vi "Measurement UI.vi"() -> ()   [LabVIEW 2021, in "Single Point_Channel Ganging_UI.lvlib"]
uses:
  Single Point_Channel Ganging_UI.lvlib
  shared/UI/controls/view.ctl
panel:
  in  "MeasGraphs":enum32{"Results", "Hidden Controls"}(tab)
  in  "Current v/s Time":string="CURRENT v/s TIME"
  in  "Voltage v/s Time":string="VOLTAGE v/s TIME"
  in  "view current legend":T1
  in  "view voltage legend":T1
  out "CurrentGraph":waveform(dbl)[](graph) caption="AC"
  out "VoltageGraph":waveform(dbl)[](graph) caption="AC"
  in  "Mode of operation":T2(ring)
  out "Maximum values":dbl[](array[numeric])
  out "Minimum values":dbl[](array[numeric])
  out "Mean values":dbl[](array[numeric])
  in  "Load resource names":string[](array[string])
  in  "Power ON/Source resource names":string[](array[string])
  out "Ganged load currents":dbl[](array[numeric])
  out "Ganged load voltages":dbl[](array[numeric])
  out "Ganged source currents":dbl[](array[numeric])
  out "Ganged source voltages":dbl[](array[numeric])
  out "Load currents":dbl[](array[numeric])
  out "Load voltages":dbl[](array[numeric])
  out "Source currents":dbl[](array[numeric])
  out "Source voltages":dbl[](array[numeric])
  out "dt":dbl[](array[numeric])
  out "Meas Table":string[][](table)=[["Source Voltage (V)"], ["Source Current (A)"], ["Load Voltage (V)"], ["Load Current (A)"]]
  in  "ModeOfConfiguration":T3(tab)
  in  "DEVICE POWER":bool=TRUE
  out "Status":string
  in  "Load config power on":string="Load Config"
  in  "POWERON/OFFLOADResourceNames":refnum<k15>[](array[refnum]) caption="RESOURCE NAMES\n(Single/Master & Slave)"
  in  "Source config power on":string="Source Config"
  in  "POWERON/OFFSOURCEResourceNames":refnum<k15>[](array[refnum]) caption="RESOURCE NAMES\n(Single/Master & Slave)"
  in  "Power on/off source sense":i32(ring)=1009 caption="SENSE" items=["Local"=1008, "Remote"=1009]
  in  "Power on/off Source voltage/current limit range":dbl=20.0 caption="CURRENT LIMIT" format="%#_6pA"
  in  "Power on/off Source voltage/current level":dbl=6.0 caption="VOLTAGE LEVEL" format="%#_6pV"
  in  "Power on/off source system configuration":enum32{"Series", "Parallel"}(ring)=enum."Parallel" caption="SYSTEM CONFIG"
  in  "Power on/off output function":i32(ring)=1006 caption="OUTPUT FUNCTION" items=["DC Voltage"=1006, "DC Current"=1007]
  out "Eload status":string
  in  "MeasConfigurations":T4(tab)=enum."Source Config"
  in  "Measurement timeout":dbl=1.0 caption="MEASUREMENT TIMEOUT" format="%.3ps"
  in  "Aperture time":dbl=0.01666 caption="APERTURE TIME" format="%.3ps"
  in  "Measurement duration":dbl=1.0 caption="MEASUREMENT DURATION" format="%.3ps"
  in  "Source voltage/current compensation frequency":dbl(slide)=3530.0 caption="COMP. FREQUENCY" scale=50.0..1000000.0 scale format="%#_6pHz"
  in  "Source voltage/current pole-zero ratio":dbl(slide)=2.0 caption="POLE-ZERO RATIO" scale=0.0625..16.0
  in  "Source voltage/current gain bandwidth":dbl(slide)=2000.0 caption="GAIN BANDWIDTH" scale=10.0..1000000.0 scale format="%#_6pHz"
  in  "Source enable/disable":bool=TRUE caption="Source Enable/Disable"
  in  "PPSResourceNames":refnum<k15>[](array[refnum]) caption="RESOURCE NAMES\n(Single/Master & Slave)"
  in  "Source transient response":i32(ring)=1038 caption="TRANSIENT RESPONSE" items=["Slow"=1041, "Normal"=1038, "Fast"=1039, "Custom"=1042]
  in  "Power ON/Source sense":i32(ring)=1009 caption="SENSE" items=["Local"=1008, "Remote"=1009]
  in  "Source voltage/current level range":dbl=20.0 caption="VOLTAGE LEVEL RANGE" format="%#_6pV"
  in  "Power ON/Source voltage/current level":dbl=6.0 caption="VOLTAGE LEVEL" format="%#_6pV"
  in  "Source current/voltage limit high":dbl=25.0 caption="CURRENT LIMIT/LIMIT HIGH" format="%#_6pA"
  in  "Power ON/Source current/voltage limit range":dbl=25.0 caption="CURRENT LIMIT RANGE" format="%#_6pA"
  in  "Source limit symmetry":enum32{"Symmetric", "Asymmetric"}(ring)=enum."Asymmetric" caption="LIMIT SYMMETRY"
  in  "Source current/voltage limit low":dbl=-0.6 caption="CURRENT LIMIT LOW" format="%#_6pA"
  in  "Power ON/Source system configuration":enum32{"Series", "Parallel"}(ring)=enum."Parallel" caption="SYSTEM CONFIG"
  in  "Source compliance":string="Compliance"
  in  "Source sourceadapt":string="SourceAdapt"
  in  "Power ON/Source output function":i32(ring)=1006 caption="OUTPUT FUNCTION" items=["DC Voltage"=1006, "DC Current"=1007]
  in  "Load voltage/current compensation frequency":dbl(slide)=3530.0 caption="COMP. FREQUENCY" scale=50.0..1000000.0 scale format="%#_6pHz"
  in  "Load voltage/current pole-zero ratio":dbl(slide)=2.0 caption="POLE-ZERO RATIO" scale=0.0625..16.0
  in  "Load voltage/current gain bandwidth":dbl(slide)=2000.0 caption="GAIN BANDWIDTH" scale=10.0..1000000.0 scale format="%#_6pHz"
  in  "Load device voltage/current rating":dbl=30.0 caption="MAX CURRENT PER LOAD" format="%#_6pA"
  in  "Load sourceadapt":string="SourceAdapt"
  in  "Load compliance":string="Compliance"
  in  "Load system configuration":enum32{"Series", "Parallel"}(ring)=enum."Parallel" caption="SYSTEM CONFIG"
  in  "Load current/voltage limit low":dbl caption="VOLTAGE  LIMIT LOW" format="%#_6pV"
  in  "Load limit symmetry":enum32{"Symmetric", "Asymmetric"}(ring) caption="LIMIT SYMMETRY"
  in  "Load current/voltage limit range":dbl=6.0 caption="VOLTAGE LIMIT RANGE" format="%#_6pV"
  in  "Load current/voltage limit high":dbl=inf caption="VOLTAGE LIMIT/LIMIT HIGH" format="%#_6p"
  in  "Load voltage/current level":dbl=2.0 caption="CURRENT LEVEL" format="%#_6pA"
  in  "Load voltage/current level range":dbl=40.0 caption="CURRENT LEVEL RANGE" format="%#_6pA"
  in  "Load sense":i32(ring)=1009 caption="SENSE" items=["Local"=1008, "Remote"=1009]
  in  "Load transient response":i32(ring)=1038 caption="TRANSIENT RESPONSE" items=["Slow"=1041, "Normal"=1038, "Fast"=1039, "Custom"=1042]
  in  "Load output function":i32(ring)=1007 caption="OUTPUT FUNCTION" items=["DC Voltage"=1006, "DC Current"=1007]
  in  "Load enable/disable":bool=TRUE caption="Load Enable/Disable"
  in  "LoadResourceNames":refnum<k15>[](array[refnum]) caption="RESOURCE NAMES\n(Single/Master & Slave)"
  # "V"
  # "I"
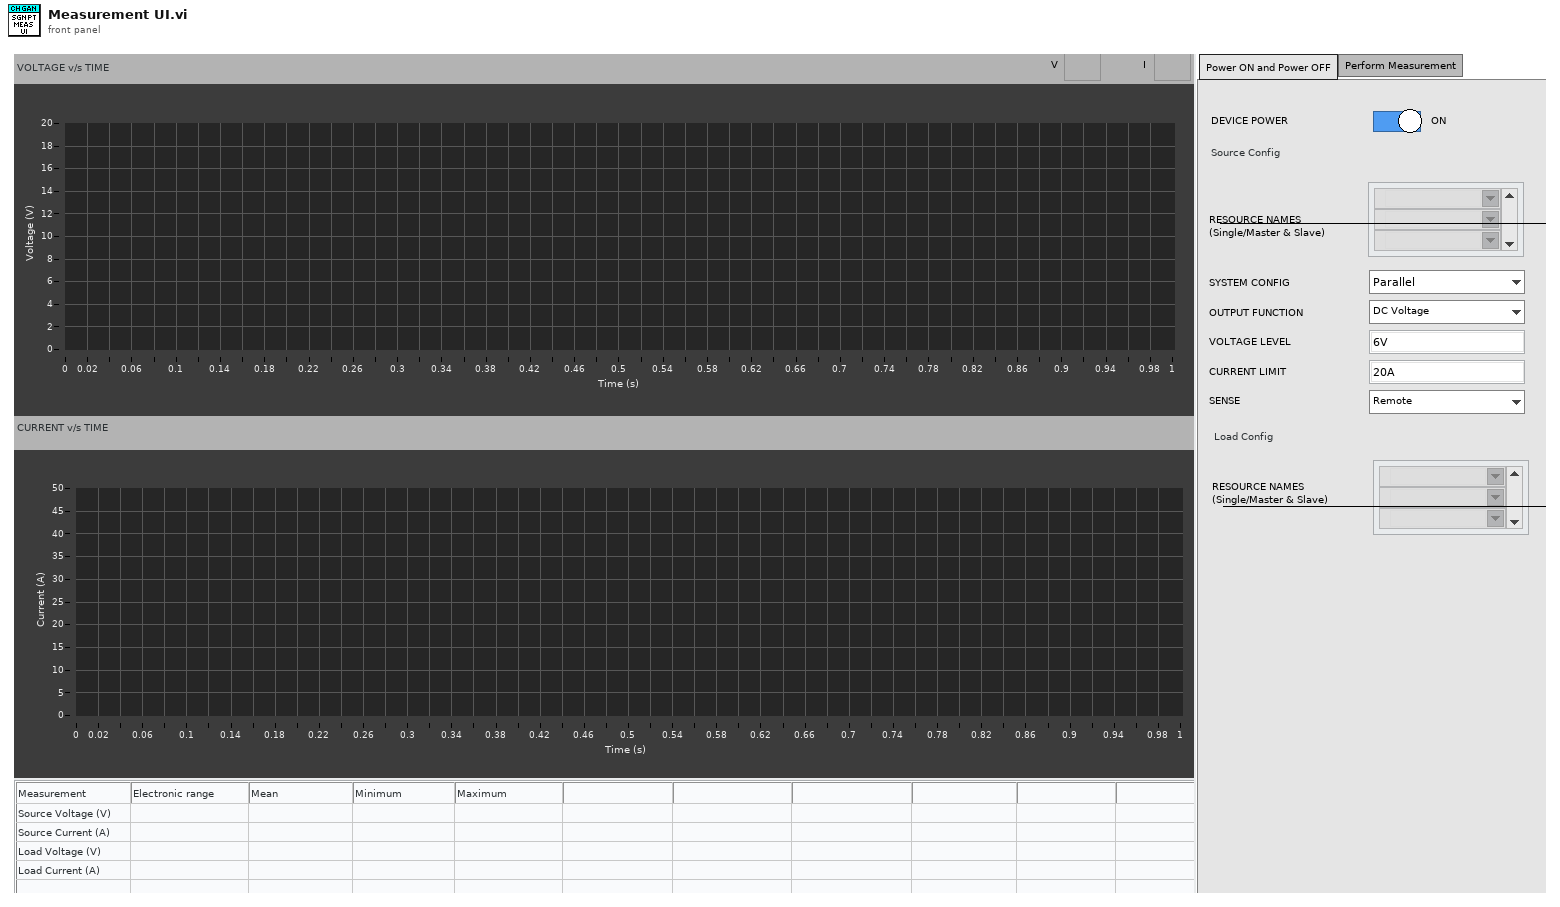
[diagram p1: front panel]
types:
  T1 = typedef "view.ctl" = bool
  T2 = enum32{"Power on the DUT", "Perform measurement", "Power off the DUT"}
  T3 = enum32{"Power ON and Power OFF", "Perform Measurement"}
  T4 = enum32{"Timings", "Source Config", "Load Config"}
  T5 = enum8{"Enabled", "Disabled", "Disabled and Grayed Out"}
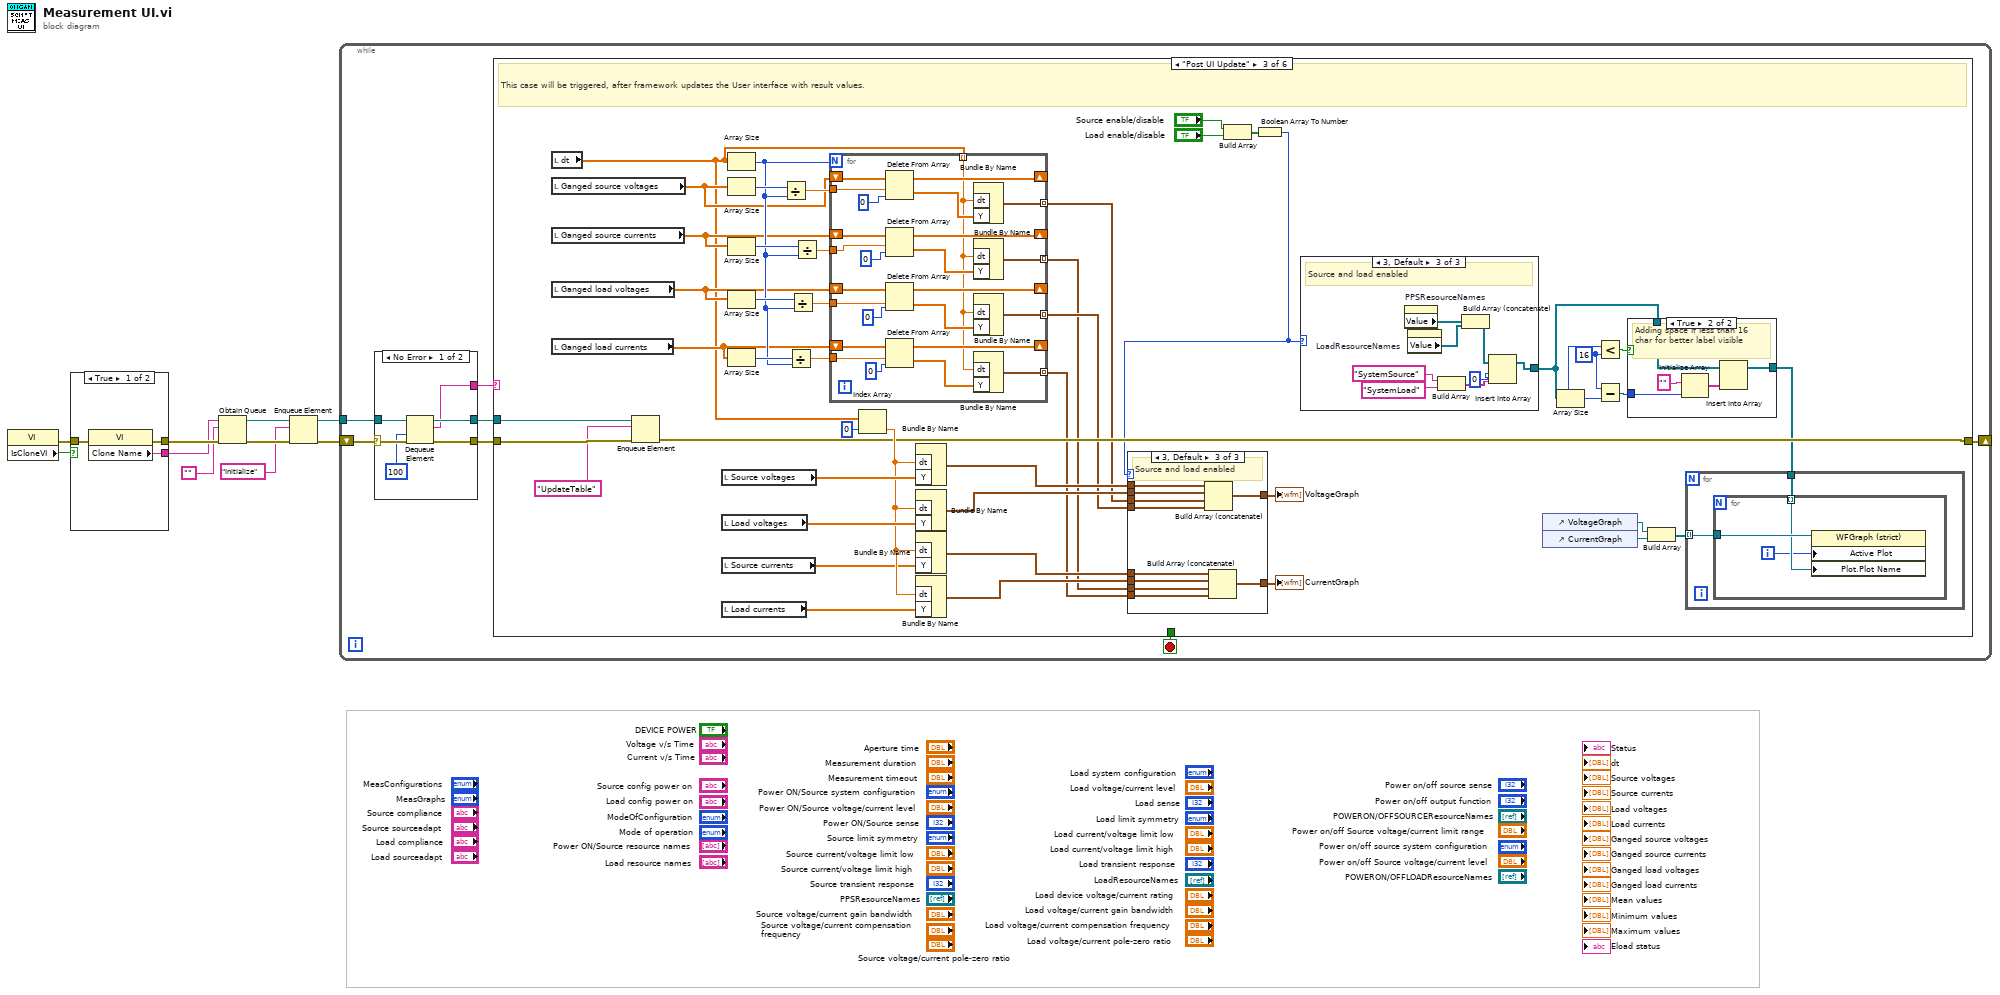
[diagram p0: block diagram]
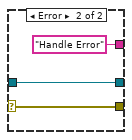
[diagram p2: hidden frame]
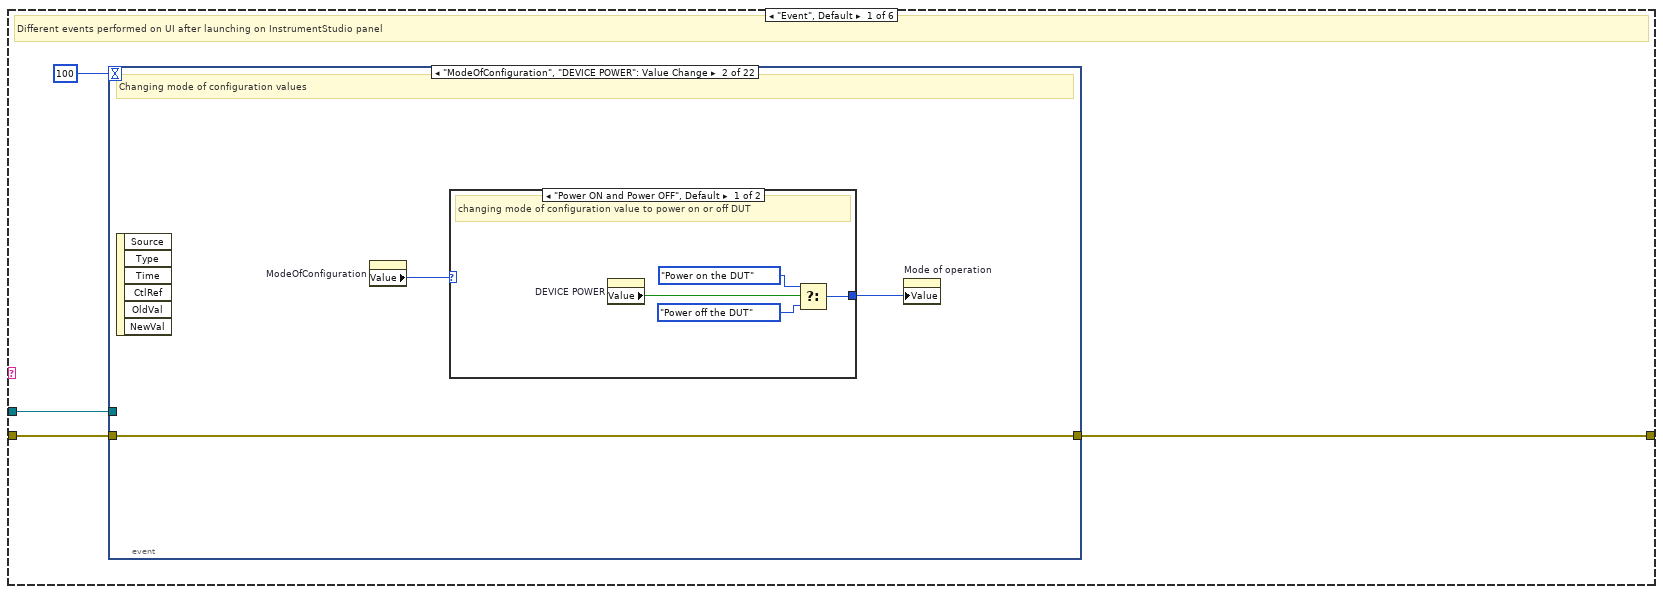
[diagram p3: hidden frame]
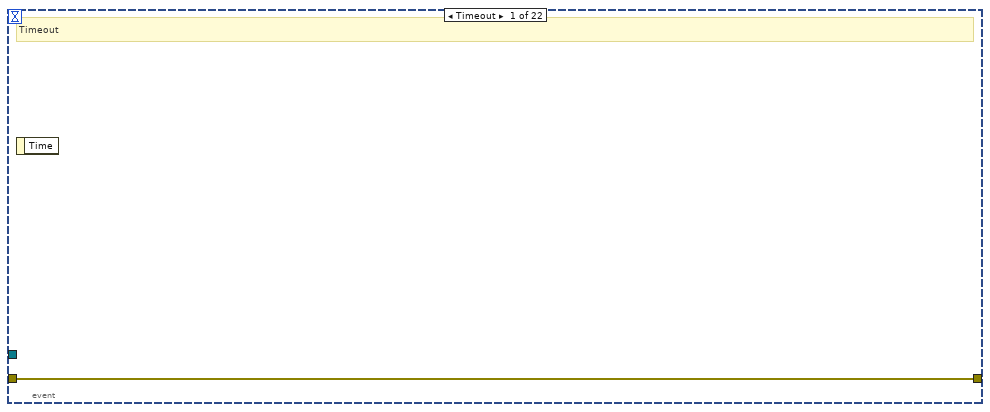
[diagram p4: hidden frame]
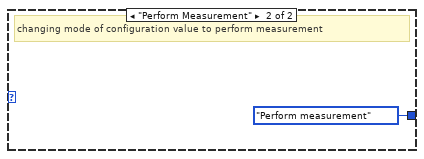
[diagram p5: hidden frame]
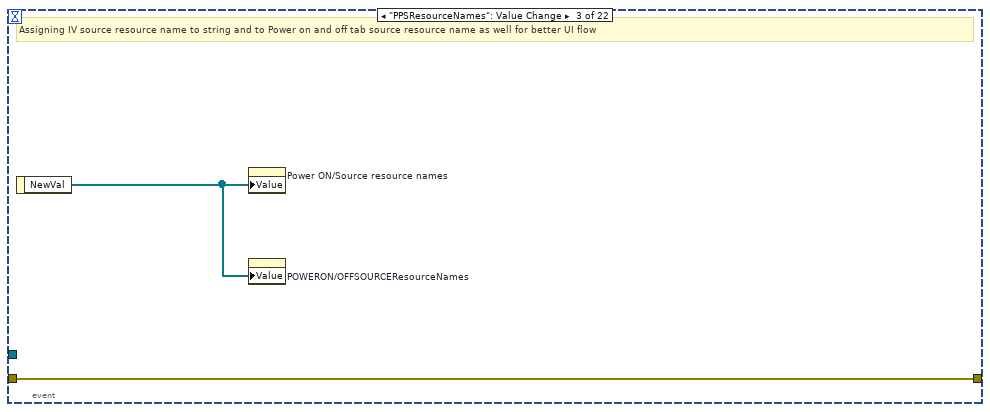
[diagram p6: hidden frame]
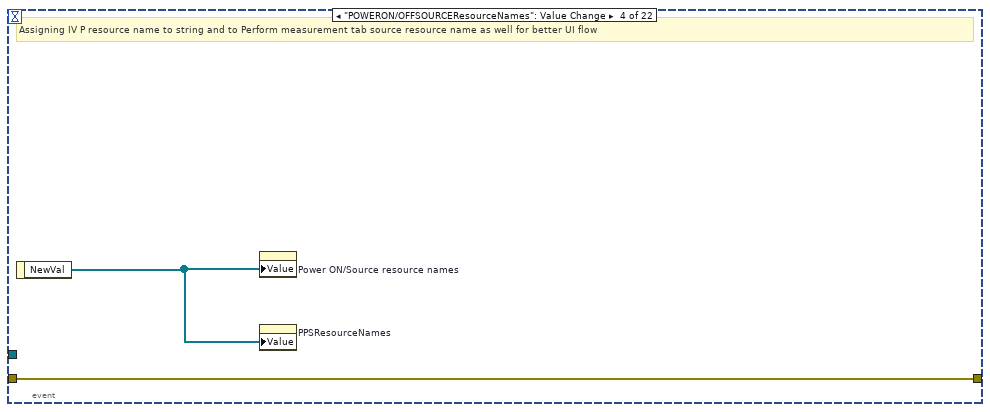
[diagram p7: hidden frame]
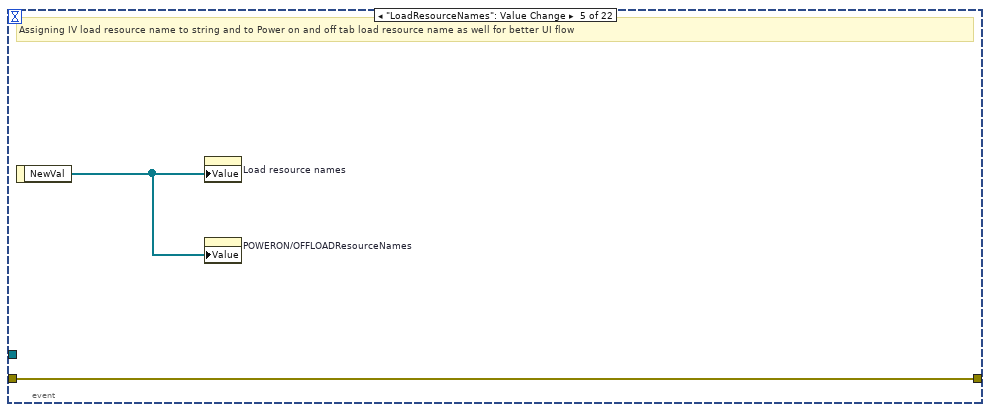
[diagram p8: hidden frame]
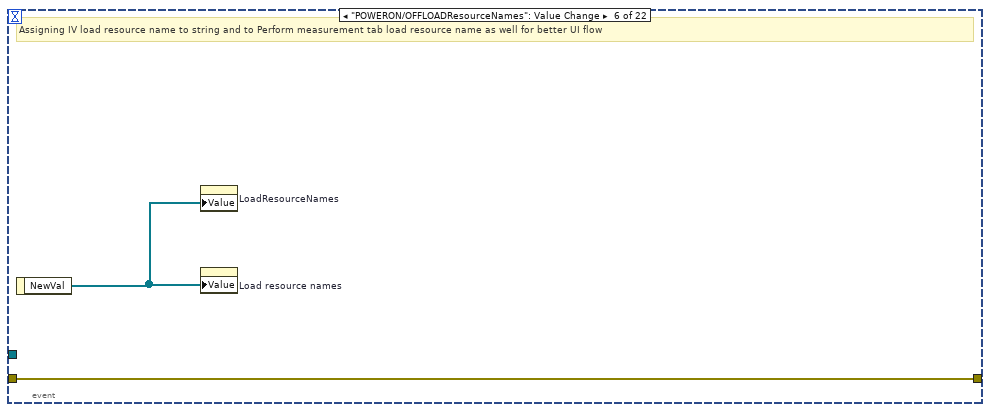
[diagram p9: hidden frame]
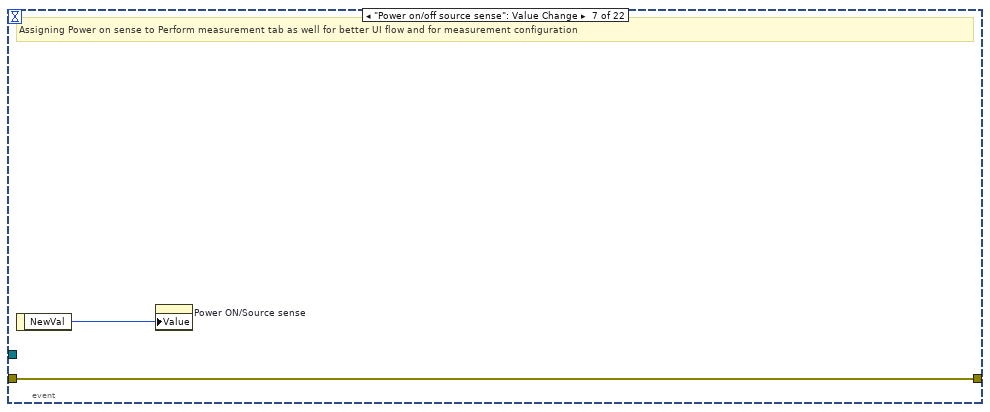
[diagram p10: hidden frame]
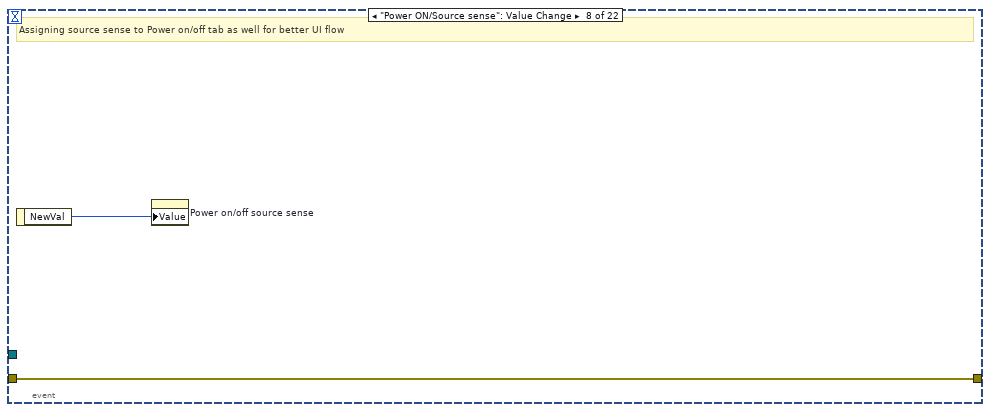
[diagram p11: hidden frame]
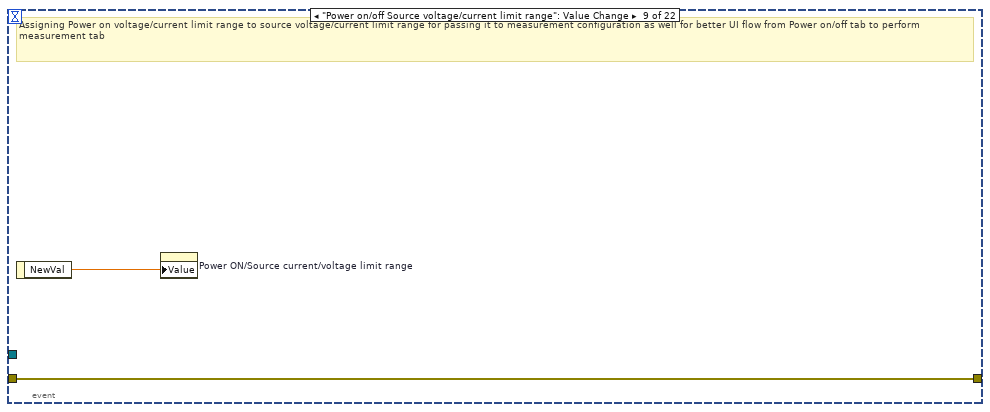
[diagram p12: hidden frame]
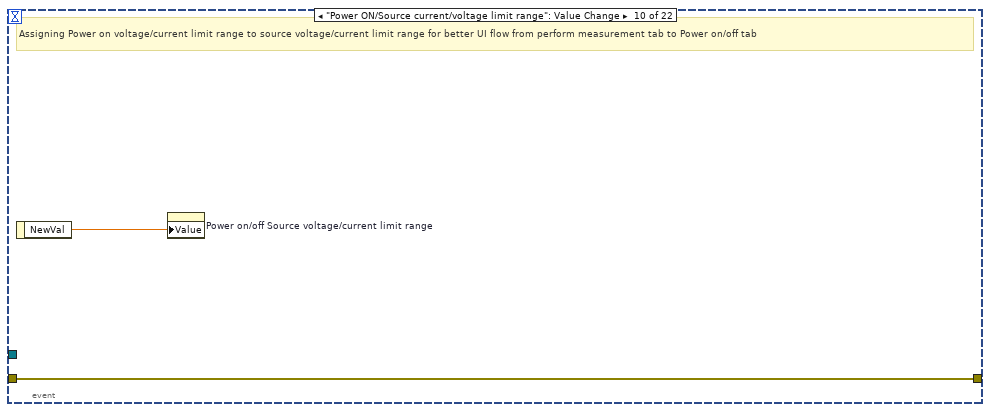
[diagram p13: hidden frame]
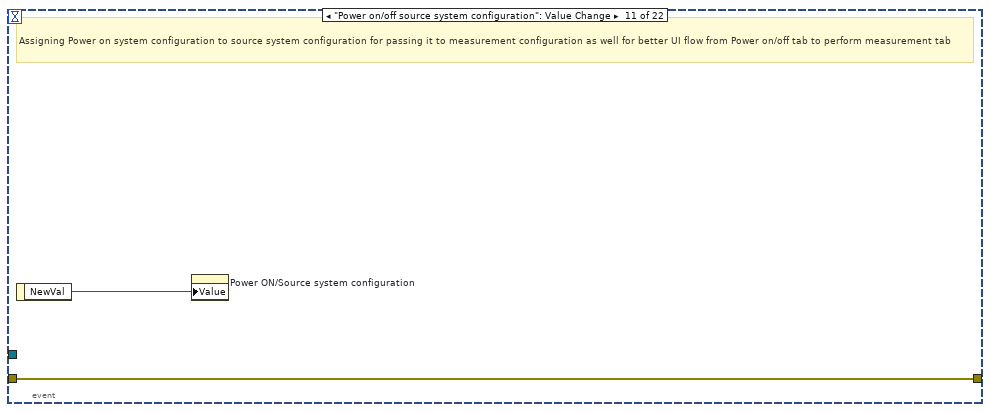
[diagram p14: hidden frame]
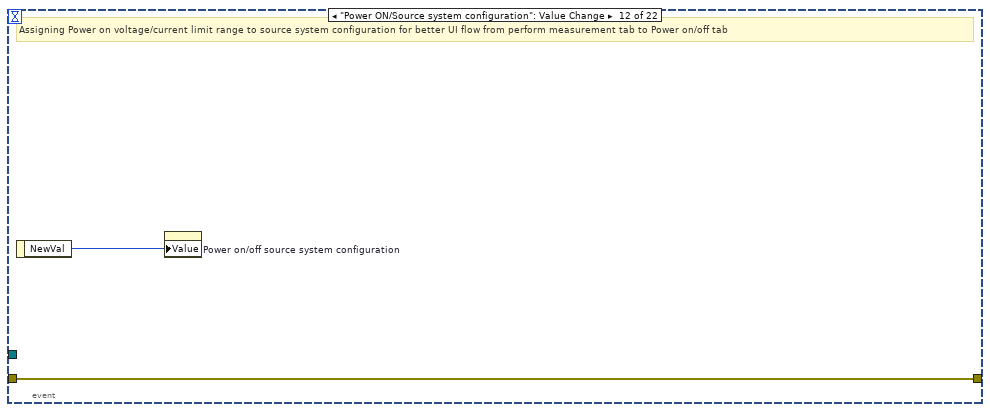
[diagram p15: hidden frame]
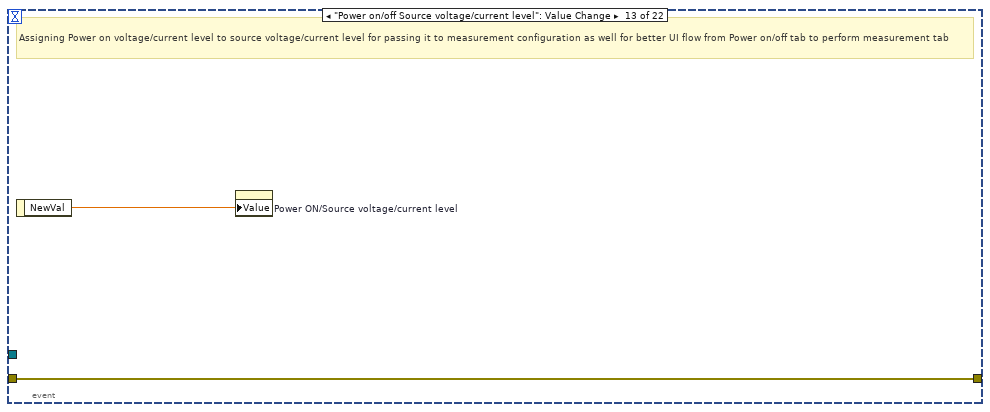
[diagram p16: hidden frame]
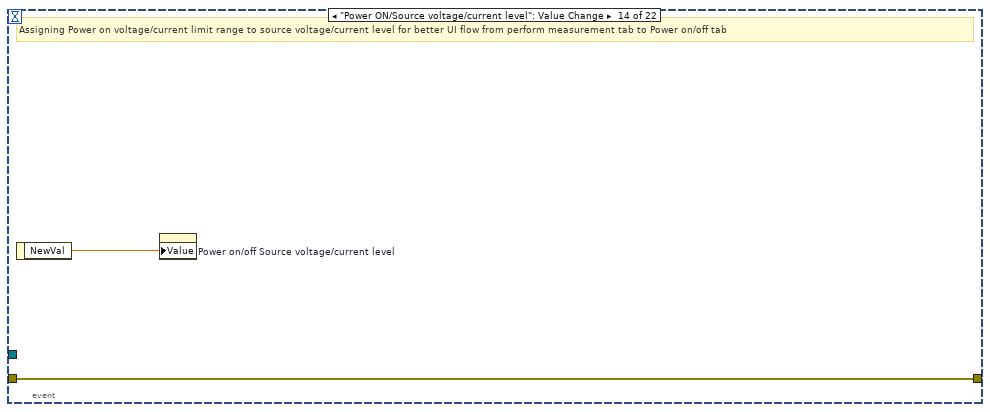
[diagram p17: hidden frame]
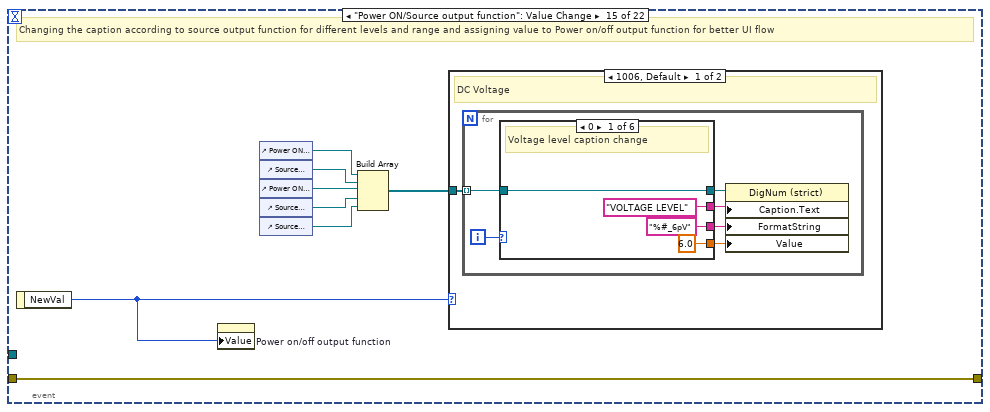
[diagram p18: hidden frame]
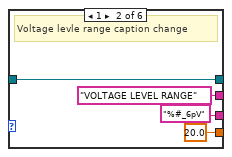
[diagram p19: hidden frame]
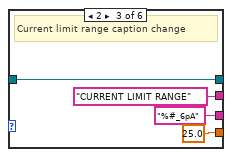
[diagram p20: hidden frame]
diagram:
  n1 = property class="VI"() -> (error out=w1:errorcluster, "IsCloneVI"=w2:bool)  [unwired: 2 in, 1 out]
  n2 = case shown="True" w2 {
    tunnel: [w13 w16] -> w10
    tunnel: [w12 w15] -> w9
    tunnel: w1 -> [w11 w14]
    frame True {
      n3 = property class="VI"(error in=w11) -> (error out=w13:errorcluster, "Clone Name"=w12:string)  [unwired: 1 in, 1 out]
    }
    frame False {
      n4 = property class="VI"(error in=w14) -> (error out=w16:errorcluster, "Name"=w15:string)  [unwired: 1 in, 1 out]
    }
  }
  n5 = Obtain Queue(name (unnamed)=w9, element data type="", error in (no error)=w10) -> (queue out=w6:refnum<queue>, error out=w8:errorcluster)  [unwired: 2 in, 1 out]
  n6 = Enqueue Element(queue=w6, element="Initialize", error in (no error)=w8) -> (queue out=w5:refnum<queue>, error out=w7:errorcluster)  [unwired: 1 in, 1 out]
  n7 = while {
    shift-right: [w18] -> _
    shift-left: w7 -> [w23]
    tunnel: w5 -> [w21]
    stop <- w17 stop-if-true
    n8 = case shown="No Error" w23 {
      selector: w23 -> [w29 w32]
      tunnel: [w28 w32] -> w22
      tunnel: w21 -> [w27 w31]
      tunnel: [w26 w31] -> w20
      tunnel: [w25 "Handle Error"] -> w19
      frame No Error {
        n9 = Dequeue Element(queue=w27, timeout in ms (-1)=100, error in (no error)=w29) -> (queue out=w26:refnum<queue>, element=w25:string, error out=w28:errorcluster)  [unwired: 1 out]
      }
      frame Error {
      }
    }
    n10 = case shown="\"Post UI Update\"" w19 {
      tunnel: w22 -> [w35 w281 w304 w431 w463 w464]
      tunnel: w20 -> [w33 _ w303 _ w461 _]
      tunnel: [w36 w281 w305 w431 w458 w464] -> w18
      tunnel: [_ _ _ _ TRUE _] -> w17
      frame "Event", Default {
        # "Different events performed on UI after launching on InstrumentStudio panel"
        n11 = event shown="[1] \"ModeOfConfiguration\", \"DEVICE POWER\": Value Change" {
          selector: _ -> [_ _ _ _ _ _ _ _ _ _ _ _ _ _ _ _ _ _ _ _ _ _]
          dyn-events: _ -> [_ _ _ _ _ _ _ _ _ _ _ _ _ _ _ _ _ _ _ _ _ _]
          timeout: 100 -> [_ _ _ _ _ _ _ _ _ _ _ _ _ _ _ _ _ _ _ _ _ _]
          tunnel: [w37 w38 w47 w48 w51 w52 w54 w56 w58 w60 w62 w65 w66 w69 w70 w136 w179 w244 w249 w252 w265 w278] -> w36
          tunnel: w35 -> [w37 w38 w47 w48 w51 w52 w54 w56 w58 w60 w62 w65 w66 w69 w70 w136 w179 w244 w249 w253 w266 w279]
          tunnel: w33 -> [_ _ _ _ _ _ _ _ _ _ _ _ _ _ _ _ _ _ _ _ _ w277]
          event Timeout {
            # "Timeout"
            n12 = event-data() -> ()  [unwired: 1 in, 1 out]
          }
          event "ModeOfConfiguration", "DEVICE POWER": Value Change {
            # "Changing mode of configuration values"
            n13 = event-data() -> ()  [unwired: 1 in, 6 out]
            n14 = property on="ModeOfConfiguration" class="TabCtl (strict)"() -> ("Value"=w40:T3)  [unwired: 2 in, 2 out]
            n15 = case shown="\"Power ON and Power OFF\", Default" w40 {
              tunnel: [w42 T2."Perform measurement" ("Mode of operation")] -> w39
              frame "Power ON and Power OFF", Default {
                # "changing mode of configuration value to power on or off DUT"
                n16 = property on="DEVICE POWER" class="Bool (strict)"() -> ("Value"=w41:bool)  [unwired: 2 in, 2 out]
                n17 = Select(t=T2."Power on the DUT" ("Mode of operation"), s=w41, f=T2."Power off the DUT" ("Mode of operation")) -> (s? t:f=w42:T2)
              }
              frame "Perform Measurement" {
                # "changing mode of configuration value to perform measurement"
              }
            }
            n18 = property on="Mode of operation" class="Enum (strict)"("Value"=w39) -> ()  [unwired: 2 in, 2 out]
          }
          event "PPSResourceNames": Value Change {
            # "Assigning IV source resource name to string and to Power on and off tab source resource name as well for better UI flow"
            n19 = event-data() -> ("NewVal"=w46:refnum<k15>[])  [unwired: 1 in]
            n20 = property on="Power ON/Source resource names" class="Arr (strict)"("Value"=w46) -> ()  [unwired: 2 in, 2 out]
            n21 = property on="POWERON/OFFSOURCEResourceNames" class="Arr (strict)"("Value"=w46) -> ()  [unwired: 2 in, 2 out]
          }
          event "POWERON/OFFSOURCEResourceNames": Value Change {
            # "Assigning IV P resource name to string and to Perform measurement tab source resource name as well for better UI flow"
            n22 = event-data() -> ("NewVal"=w49:refnum<k15>[])  [unwired: 1 in]
            n23 = property on="Power ON/Source resource names" class="Arr (strict)"("Value"=w49) -> ()  [unwired: 2 in, 2 out]
            n24 = property on="PPSResourceNames" class="Arr (strict)"("Value"=w49) -> ()  [unwired: 2 in, 2 out]
          }
          event "LoadResourceNames": Value Change {
            # "Assigning IV load resource name to string and to Power on and off tab load resource name as well for better UI flow"
            n25 = event-data() -> ("NewVal"=w50:refnum<k15>[])  [unwired: 1 in]
            n26 = property on="Load resource names" class="Arr (strict)"("Value"=w50) -> ()  [unwired: 2 in, 2 out]
            n27 = property on="POWERON/OFFLOADResourceNames" class="Arr (strict)"("Value"=w50) -> ()  [unwired: 2 in, 2 out]
          }
          event "POWERON/OFFLOADResourceNames": Value Change {
            # "Assigning IV load resource name to string and to Perform measurement tab load resource name as well for better UI flow"
            n28 = event-data() -> ("NewVal"=w53:refnum<k15>[])  [unwired: 1 in]
            n29 = property on="LoadResourceNames" class="Arr (strict)"("Value"=w53) -> ()  [unwired: 2 in, 2 out]
            n30 = property on="Load resource names" class="Arr (strict)"("Value"=w53) -> ()  [unwired: 2 in, 2 out]
          }
          event "Power on/off source sense": Value Change {
            # "Assigning Power on sense to Perform measurement tab as well for better UI flow and for measurement configuration"
            n31 = event-data() -> ("NewVal"=w55:i32)  [unwired: 1 in]
            n32 = property on="Power ON/Source sense" class="Ring (strict)"("Value"=w55) -> ()  [unwired: 2 in, 2 out]
          }
          event "Power ON/Source sense": Value Change {
            # "Assigning source sense to Power on/off tab as well for better UI flow"
            n33 = event-data() -> ("NewVal"=w57:i32)  [unwired: 1 in]
            n34 = property on="Power on/off source sense" class="Ring (strict)"("Value"=w57) -> ()  [unwired: 2 in, 2 out]
          }
          event "Power on/off Source voltage/current limit range": Value Change {
            # "Assigning Power on voltage/current limit range to source voltage/current limit range for passing it to measurement configuration as well for better UI flow from Power on/off tab to perform measurement tab"
            n35 = event-data() -> ("NewVal"=w59:dbl)  [unwired: 1 in]
            n36 = property on="Power ON/Source current/voltage limit range" class="DigNum (strict)"("Value"=w59) -> ()  [unwired: 2 in, 2 out]
          }
          event "Power ON/Source current/voltage limit range": Value Change {
            # "Assigning Power on voltage/current limit range to source voltage/current limit range for better UI flow from perform measurement tab to Power on/off tab"
            n37 = event-data() -> ("NewVal"=w61:dbl)  [unwired: 1 in]
            n38 = property on="Power on/off Source voltage/current limit range" class="DigNum (strict)"("Value"=w61) -> ()  [unwired: 2 in, 2 out]
          }
          event "Power on/off source system configuration": Value Change {
            # "Assigning Power on system configuration to source system configuration for passing it to measurement configuration as well for better UI flow from Power on/off tab to perform measurement tab"
            n39 = event-data() -> ("NewVal"=w63:enum32{"Series", "Parallel"})  [unwired: 1 in]
            n40 = property on="Power ON/Source system configuration" class="Enum (strict)"("Value"=w63) -> ()  [unwired: 2 in, 2 out]
          }
          event "Power ON/Source system configuration": Value Change {
            # "Assigning Power on voltage/current limit range to source system configuration for better UI flow from perform measurement tab to Power on/off tab"
            n41 = event-data() -> ("NewVal"=w64:enum32{"Series", "Parallel"})  [unwired: 1 in]
            n42 = property on="Power on/off source system configuration" class="Enum (strict)"("Value"=w64) -> ()  [unwired: 2 in, 2 out]
          }
          event "Power on/off Source voltage/current level": Value Change {
            # "Assigning Power on voltage/current level to source voltage/current level for passing it to measurement configuration as well for better UI flow from Power on/off tab to perform measurement tab"
            n43 = event-data() -> ("NewVal"=w67:dbl)  [unwired: 1 in]
            n44 = property on="Power ON/Source voltage/current level" class="DigNum (strict)"("Value"=w67) -> ()  [unwired: 2 in, 2 out]
          }
          event "Power ON/Source voltage/current level": Value Change {
            # "Assigning Power on voltage/current limit range to source voltage/current level for better UI flow from perform measurement tab to Power on/off tab"
            n45 = event-data() -> ("NewVal"=w68:dbl)  [unwired: 1 in]
            n46 = property on="Power on/off Source voltage/current level" class="DigNum (strict)"("Value"=w68) -> ()  [unwired: 2 in, 2 out]
          }
          event "Power ON/Source output function": Value Change {
            # "Changing the caption according to source output function for different levels and range and assigning value to Power on/off output function for better UI flow"
            n47 = event-data() -> ("NewVal"=w71:i32)  [unwired: 1 in]
            n48 = property on="Power on/off output function" class="Ring (strict)"("Value"=w71) -> ()  [unwired: 2 in, 2 out]
            n49 = control-ref of="Power ON/Source voltage/current level"() -> (w77:refnum<vi>)
            n50 = control-ref of="Source voltage/current level range"() -> (w76:refnum<vi>)
            n51 = control-ref of="Power ON/Source current/voltage limit range"() -> (w75:refnum<vi>)
            n52 = control-ref of="Source current/voltage limit low"() -> (w74:refnum<vi>)
            n53 = control-ref of="Source current/voltage limit high"() -> (w73:refnum<vi>)
            n54 = Build Array(w77, w76, w75, w74, w73) -> (w72:refnum<vi>[])
            n55 = case shown="1006, Default" w71 {
              tunnel: w72 -> [w78 w105]
              frame 1006, Default {
                # "DC Voltage"
                n56 = for {
                  tunnel: w78 -> [w82] mode=indexing
                  i -> [w84]
                  n57 = case shown="0" w84 {
                    tunnel: [w88 w92 w96 w99 w103 _] -> w83
                    tunnel: w82 -> [w88 w92 w96 w99 w103 _]
                    tunnel: ["VOLTAGE LEVEL" ("Caption.Text") "VOLTAGE LEVEL RANGE" ("Caption.Text") "CURRENT LIMIT RANGE" ("Caption.Text") "CURRENT LIMIT LOW" ("Caption.Text") "CURRENT LIMIT/LIMIT HIGH" ("Caption.Text") _] -> w81
                    tunnel: ["%#_6pV" ("Format String") "%#_6pV" ("Format String") "%#_6pA" ("Format String") "%#_6pA" ("Format String") "%#_6pA" ("Format String") _] -> w80
                    tunnel: [6.0 ("Value") 20.0 ("Value") 25.0 ("Value") -0.6 ("Value") 25.0 ("Value") _] -> w79
                    frame 0 {
                      # "Voltage level caption change"
                    }
                    frame 1 {
                      # "Voltage levle range caption change"
                    }
                    frame 2 {
                      # "Current limit range caption change"
                    }
                    frame 3 {
                      # "Current limit low caption change"
                    }
                    frame 4 {
                      # "Current limit/limit high caption change"
                    }
                    frame Default {
                    }
                  }
                  n58 = property class="DigNum (strict)"(reference=w83, "Caption.Text"=w81, "FormatString"=w80, "Value"=w79) -> ()  [unwired: 1 in, 2 out]
                }
              }
              frame 1007 {
                # "DC Current"
                n59 = for {
                  tunnel: w105 -> [w109] mode=indexing
                  i -> [w111]
                  n60 = case shown="0" w111 {
                    tunnel: [w115 w119 w123 w126 w130 _] -> w110
                    tunnel: w109 -> [w115 w119 w123 w126 w130 _]
                    tunnel: ["CURRENT LEVEL" ("Caption.Text") "CURRENT LEVEL RANGE" ("Caption.Text") "VOLTAGE LIMIT RANGE" ("Caption.Text") "VOLTAGE LIMIT LOW" ("Caption.Text") "VOLTAGE LIMIT/LIMIT HIGH" ("Caption.Text") _] -> w108
                    tunnel: ["%#_6pA" ("Format String") "%#_6pA" ("Format String") "%#_6pV" ("Format String") "%#_6pV" ("Format String") "%#_6pV" ("Format String") _] -> w107
                    tunnel: [1.0 ("Value") 25.0 ("Value") 20.0 ("Value") -0.6 ("Value") 20.0 ("Value") _] -> w106
                    frame 0 {
                      # "Current level caption change"
                    }
                    frame 1 {
                      # "Current level range caption change"
                    }
                    frame 2 {
                      # "Voltage limit range caption change"
                    }
                    frame 3 {
                      # "Voltage limit low caption change"
                    }
                    frame 4 {
                      # "Voltage limit/limit high caption change"
                    }
                    frame Default {
                    }
                  }
                  n61 = property class="DigNum (strict)"(reference=w110, "Caption.Text"=w108, "FormatString"=w107, "Value"=w106) -> ()  [unwired: 1 in, 2 out]
                }
              }
            }
          }
          event "Power on/off output function": Value Change {
            # "Assigning Power on output function to source output function for passing it to measurement configuration as well for better UI flow"
            n62 = event-data() -> ("NewVal"=w135:i32)  [unwired: 1 in]
            n63 = property on="Power ON/Source output function" class="Ring (strict)"("Value"=w135) -> ()  [unwired: 2 in, 2 out]
            n64 = control-ref of="Power on/off Source voltage/current limit range"() -> (w133:refnum<vi>)
            n65 = control-ref of="Power on/off Source voltage/current level"() -> (w134:refnum<vi>)
            n66 = Build Array(w133, w134) -> (w132:refnum<vi>[])
            n67 = case shown="1007" w135 {
              tunnel: w132 -> [w137 w152]
              frame 1006, Default {
                # "DC Voltage"
                n68 = for {
                  tunnel: w137 -> [w141] mode=indexing
                  i -> [w143]
                  n69 = case shown="0" w143 {
                    tunnel: [w147 w151 _] -> w142
                    tunnel: w141 -> [w147 w151 _]
                    tunnel: ["VOLTAGE LEVEL" ("Caption.Text") "CURRENT LIMIT RANGE" ("Caption.Text") _] -> w140
                    tunnel: ["%#_6pV" ("Format String") "%#_6pA" ("Format String") _] -> w139
                    tunnel: [6.0 ("Value") 25.0 ("Value") _] -> w138
                    frame 0 {
                      # "Voltage level range caption change"
                    }
                    frame 1 {
                      # "Current limit range caption change"
                    }
                    frame Default {
                    }
                  }
                  n70 = property class="DigNum (strict)"(reference=w142, "Caption.Text"=w140, "FormatString"=w139, "Value"=w138) -> ()  [unwired: 1 in, 2 out]
                }
              }
              frame 1007 {
                # "DC Current"
                n71 = for {
                  tunnel: w152 -> [w156] mode=indexing
                  i -> [w158]
                  n72 = case shown="Default" w158 {
                    tunnel: [w162 w166 w170 w173 w177 _] -> w157
                    tunnel: w156 -> [w162 w166 w170 w173 w177 _]
                    tunnel: ["CURRENT LEVEL" ("Caption.Text") "CURRENT LEVEL RANGE" ("Caption.Text") "VOLTAGE LIMIT RANGE" ("Caption.Text") "VOLTAGE  LIMIT LOW" ("Caption.Text") "VOLTAGE LIMIT/LIMIT HIGH" ("Caption.Text") _] -> w155
                    tunnel: ["%#_6pA" ("Format String") "%#_6pA" ("Format String") "%#_6pV" ("Format String") "%#_6pV" ("Format String") "%#_6pV" ("Format String") _] -> w154
                    tunnel: [1.0 ("Value") 25.0 ("Value") 20.0 ("Value") -0.6 ("Value") 20.0 ("Value") _] -> w153
                    frame 0 {
                      # "Current level caption change"
                    }
                    frame 1 {
                      # "Voltage limit range caption change"
                    }
                    frame 2 {
                    }
                    frame 3 {
                    }
                    frame 4 {
                    }
                    frame Default {
                    }
                  }
                  n73 = property class="DigNum (strict)"(reference=w157, "Caption.Text"=w155, "FormatString"=w154, "Value"=w153) -> ()  [unwired: 1 in, 2 out]
                }
              }
            }
          }
          event "Load output function": Value Change {
            # "Changing the caption according to source output function for different levels and range"
            n74 = event-data() -> ("NewVal"=w181:i32)  [unwired: 1 in]
            n75 = control-ref of="Load voltage/current level"() -> (w186:refnum<vi>)
            n76 = control-ref of="Load voltage/current level range"() -> (w185:refnum<vi>)
            n77 = control-ref of="Load current/voltage limit range"() -> (w184:refnum<vi>)
            n78 = control-ref of="Load current/voltage limit low"() -> (w183:refnum<vi>)
            n79 = control-ref of="Load current/voltage limit high"() -> (w182:refnum<vi>)
            n80 = Build Array(w186, w185, w184, w183, w182) -> (w180:refnum<vi>[])
            n81 = case shown="1006" w181 {
              tunnel: w180 -> [w187 w214]
              frame 1006 {
                # "DC Voltage"
                n82 = for {
                  tunnel: w187 -> [w191] mode=indexing
                  i -> [w193]
                  n83 = case shown="0" w193 {
                    tunnel: [w197 w201 w205 w208 w212 _] -> w192
                    tunnel: w191 -> [w197 w201 w205 w208 w212 _]
                    tunnel: ["VOLTAGE LEVEL" ("Caption.Text") "VOLTAGE LEVEL RANGE" ("Caption.Text") "CURRENT LIMIT RANGE" ("Caption.Text") "CURRENT LIMIT LOW" ("Caption.Text") "CURRENT LIMIT/LIMIT HIGH" ("Caption.Text") _] -> w190
                    tunnel: ["%#_6pV" ("Format String") "%#_6pV" ("Format String") "%#_6pA" ("Format String") "%#_6pA" ("Format String") "%#_6pA" ("Format String") _] -> w189
                    tunnel: [3.3 ("Value") 6.0 ("Value") 40.0 ("Value") 0.0 ("Value") 40.0 ("Value") _] -> w188
                    frame 0 {
                      # "Voltage level caption change"
                    }
                    frame 1 {
                      # "Voltage level range caption change"
                    }
                    frame 2 {
                      # "Current limit range caption change"
                    }
                    frame 3 {
                      # "Current limit low caption change"
                    }
                    frame 4 {
                      # "Current limit/limit high caption change"
                    }
                    frame Default {
                    }
                  }
                  n84 = property class="DigNum (strict)"(reference=w192, "Caption.Text"=w190, "FormatString"=w189, "Value"=w188) -> ()  [unwired: 1 in, 2 out]
                }
              }
              frame 1007, Default {
                # "DC Current"
                n85 = for {
                  tunnel: w214 -> [w218] mode=indexing
                  i -> [w220]
                  n86 = case shown="0" w220 {
                    tunnel: [w224 w228 w232 w235 w240 _] -> w219
                    tunnel: w218 -> [w224 w228 w232 w235 w240 _]
                    tunnel: ["CURRENT LEVEL" ("Caption.Text") "CURRENT LEVEL RANGE" ("Caption.Text") "VOLTAGE LIMIT RANGE" ("Caption.Text") "VOLTAGE LIMIT LOW" ("Caption.Text") "VOLTAGE LIMIT/LIMIT HIGH" ("Caption.Text") _] -> w217
                    tunnel: ["%#_6pA" ("Format String") "%#_6pA" ("Format String") "%#_6pV" ("Format String") "%#_6pV" ("Format String") "%#_6p" ("Format String") _] -> w216
                    tunnel: [2.0 ("Value") 40.0 ("Value") 6.0 ("Value") 0.0 ("Value") w238 _] -> w215
                    frame 0 {
                      # "Current level caption change"
                    }
                    frame 1 {
                      # "current level range caption change"
                    }
                    frame 2 {
                      # "Voltage limit range caption change"
                    }
                    frame 3 {
                      # "Voltage limit low caption change"
                    }
                    frame 4 {
                      # "Voltage limit/limit high caption change"
                      n87 = Reciprocal(x=0.0) -> (1/x=w238:dbl)
                    }
                    frame Default {
                    }
                  }
                  n88 = property class="DigNum (strict)"(reference=w219, "Caption.Text"=w217, "FormatString"=w216, "Value"=w215) -> ()  [unwired: 1 in, 2 out]
                }
              }
            }
          }
          event "Source transient response": Value Change {
            # "Enabling and disabling source transient properties according to transient response"
            n89 = event-data() -> ("NewVal"=w243:i32)  [unwired: 1 in]
            n90 = case shown="1042" w243 {
              tunnel: [T5."Disabled and Grayed Out" ("Disabled") T5."Enabled" ("Disabled")] -> w242
              frame 1038, 1039, 1041, Default {
                # "Slow, Normal and Fast transient disables and grey out the following controls"
              }
              frame 1042 {
                # "Custom transient enables the following controls"
              }
            }
            n91 = property on="Source voltage/current compensation frequency" class="Slide (strict)"("DisabledEnum"=w242) -> ()  [unwired: 2 in, 2 out]
            n92 = property on="Source voltage/current pole-zero ratio" class="Slide (strict)"("DisabledEnum"=w242) -> ()  [unwired: 2 in, 2 out]
            n93 = property on="Source voltage/current gain bandwidth" class="Slide (strict)"("DisabledEnum"=w242) -> ()  [unwired: 2 in, 2 out]
          }
          event "Load transient response": Value Change {
            # "Enabling and disabling load transient properties according to transient response"
            n94 = event-data() -> ("NewVal"=w248:i32)  [unwired: 1 in]
            n95 = case shown="1042" w248 {
              tunnel: [T5."Disabled and Grayed Out" ("Disabled") T5."Enabled" ("Disabled")] -> w247
              frame 1038, 1039, 1041, Default {
                # "Slow, Normal and Fast transient disables and grey out the following controls"
              }
              frame 1042 {
                # "Custom transient enables the following controls"
              }
            }
            n96 = property on="Load voltage/current gain bandwidth" class="Slide (strict)"("DisabledEnum"=w247) -> ()  [unwired: 2 in, 2 out]
            n97 = property on="Load voltage/current gain bandwidth" class="Slide (strict)"("DisabledEnum"=w247) -> ()  [unwired: 2 in, 2 out]
            n98 = property on="Load voltage/current compensation frequency" class="Slide (strict)"("DisabledEnum"=w247) -> ()  [unwired: 2 in, 2 out]
          }
          event Value Change {
            # "Showing legends according click on view button for voltage"
            n99 = event-data() -> ("NewVal"=w254:T1)  [unwired: 1 in]
            n100 = control-ref of="VoltageGraph"() -> (w255:refnum<vi>)
            n101 = case shown="True" w254 {
              tunnel: w255 -> [w259 w263]
              tunnel: w253 -> [w258 w261]
              tunnel: [w256 w260] -> w252
              frame False {
                # "Don't view legends"
                n102 = property on="Property Node" class="WFGraph (strict)"(reference=w259, error in=w258, "Legend Visible"=FALSE ("Legend:Visible")) -> (error out=w256:errorcluster)  [unwired: 1 out]
              }
              frame True {
                w262 = TRUE ("Legend:Visible")
                # "View legends by click of button"
                n103 = property on="Property Node" class="WFGraph (strict)"(reference=w263, error in=w261, "Legend Visible"=w262, "PlotVisCheckbox"=w262) -> (error out=w260:errorcluster)  [unwired: 1 out]
              }
            }
          }
          event Value Change {
            # "Showing legends according click on view button for current"
            n104 = event-data() -> ("NewVal"=w267:T1)  [unwired: 1 in]
            n105 = control-ref of="CurrentGraph"() -> (w264:refnum<vi>)
            n106 = case shown="True" w267 {
              tunnel: w264 -> [w271 w275]
              tunnel: w266 -> [w270 w273]
              tunnel: [w268 w272] -> w265
              frame False {
                # "Don't view legends"
                n107 = property on="Property Node" class="WFGraph (strict)"(reference=w271, error in=w270, "Legend Visible"=FALSE ("Legend:Visible")) -> (error out=w268:errorcluster)  [unwired: 1 out]
              }
              frame True {
                w274 = TRUE ("Legend:Visible")
                # "View legends by click of button"
                n108 = property on="Property Node" class="WFGraph (strict)"(reference=w275, error in=w273, "Legend Visible"=w274, "PlotVisCheckbox"=w274) -> (error out=w272:errorcluster)  [unwired: 1 out]
              }
            }
          }
          event Panel Close? {
            n109 = event-data() -> ()  [unwired: 1 in, 4 out]
            n110 = Enqueue Element(queue=w277, element="Exit", error in (no error)=w279) -> (error out=w278:errorcluster)  [unwired: 1 in, 2 out]
            n111 = event-data("Discard?"=TRUE) -> ()  [unwired: 1 in, 1 out]
          }
        }
      }
      frame "Initialize" {
        # "Initialization of controls or indicator if needed"
      }
      frame "Post UI Update" {
        w290 = 16 ("y")
        # "This case will be triggered, after framework updates the User interface with result values."
        n112 = local read "dt"() -> (w313:dbl[])
        n113 = local read "Ganged source voltages"() -> (w316:dbl[])
        n114 = local read "Ganged source currents"() -> (w319:dbl[])
        n115 = local read "Ganged load voltages"() -> (w318:dbl[])
        n116 = local read "Ganged load currents"() -> (w317:dbl[])
        n117 = Enqueue Element(queue=w303, element="UpdateTable", error in (no error)=w304) -> (error out=w305:errorcluster)  [unwired: 1 in, 2 out]
        n118 = local read "Source voltages"() -> (w315:dbl[])
        n119 = local read "Load voltages"() -> (w314:dbl[])
        n120 = local read "Source currents"() -> (w310:dbl[])
        n121 = local read "Load currents"() -> (w309:dbl[])
        n122 = Array Size(array=w313) -> (size(s)=w323:i32)
        n123 = Array Size(array=w316) -> (size(s)=w325:i32)
        n124 = Array Size(array=w319) -> (size(s)=w324:i32)
        n125 = Array Size(array=w318) -> (size(s)=w327:i32)
        n126 = Array Size(array=w317) -> (size(s)=w328:i32)
        n127 = Divide(x=w325, y=w323) -> (x/y=w326:dbl)
        n128 = Divide(x=w328, y=w323) -> (x/y=w322:dbl)
        n129 = Divide(x=w327, y=w323) -> (x/y=w321:dbl)
        n130 = Divide(x=w324, y=w323) -> (x/y=w320:dbl)
        n131 = for {
          N: w323 -> [_]
          tunnel: w326 -> [w400]
          shift-right: [w401] -> _
          shift-left: w316 -> [w402]
          tunnel: [w395] -> w299 mode=indexing
          tunnel: [w394] -> w295 mode=indexing
          tunnel: [w393] -> w298 mode=indexing
          tunnel: [w392] -> w294 mode=indexing
          shift-right: [w386] -> _
          shift-left: w319 -> [w387]
          shift-right: [w384] -> _
          shift-left: w318 -> [w385]
          shift-right: [w382] -> _
          shift-left: w317 -> [w383]
          tunnel: w322 -> [w381]
          tunnel: w321 -> [w380]
          tunnel: w320 -> [w379]
          tunnel: w313 -> [w378] mode=indexing
          n132 = Delete From Array(array=w402, length=w400, index=0) -> (deleted portion=w391:dbl[], array with subset deleted=w401:dbl[])
          n133 = Delete From Array(array=w387, length=w379, index=0) -> (deleted portion=w390:dbl[], array with subset deleted=w386:dbl[])
          n134 = Delete From Array(array=w385, length=w380, index=0) -> (deleted portion=w389:dbl[], array with subset deleted=w384:dbl[])
          n135 = Delete From Array(array=w383, length=w381, index=0) -> (deleted portion=w388:dbl[], array with subset deleted=w382:dbl[])
          n136 = Bundle By Name("dt"=w378, "Y"=w391) -> (w395:waveform(dbl))  [unwired: 1 in]
          n137 = Bundle By Name("dt"=w378, "Y"=w390) -> (w394:waveform(dbl))  [unwired: 1 in]
          n138 = Bundle By Name("dt"=w378, "Y"=w389) -> (w393:waveform(dbl))  [unwired: 1 in]
          n139 = Bundle By Name("dt"=w378, "Y"=w388) -> (w392:waveform(dbl))  [unwired: 1 in]
        }
        n140 = Index Array(array=w313, index=0) -> (element=w311:dbl)
        n141 = Bundle By Name("dt"=w311, "Y"=w315) -> (w301:waveform(dbl))  [unwired: 1 in]
        n142 = Bundle By Name("dt"=w311, "Y"=w314) -> (w300:waveform(dbl))  [unwired: 1 in]
        n143 = Bundle By Name("dt"=w311, "Y"=w310) -> (w297:waveform(dbl))  [unwired: 1 in]
        n144 = Bundle By Name("dt"=w311, "Y"=w309) -> (w296:waveform(dbl))  [unwired: 1 in]
        n145 = Build Array("Source enable/disable", "Load enable/disable") -> (w285:bool[])
        n146 = Boolean Array To Number(Boolean array=w285) -> (number=w282:u32)
        n147 = case shown="3, Default" w282 {
          tunnel: w301 -> [w356 _ w372]
          tunnel: w300 -> [_ w360 w371]
          tunnel: [w354 w362 w370] -> w293
          tunnel: w296 -> [_ w358 w369]
          tunnel: w297 -> [w353 _ w368]
          tunnel: [w351 w361 w367] -> w292
          tunnel: w299 -> [w355 _ w366]
          tunnel: w298 -> [_ w359 w365]
          tunnel: w295 -> [w352 _ w364]
          tunnel: w294 -> [_ w357 w363]
          frame 1 {
            # "Source enabled"
            n148 = Build Array (concatenate)(w353, w352) -> (w351:waveform(dbl)[])
            n149 = Build Array (concatenate)(w356, w355) -> (w354:waveform(dbl)[])
          }
          frame 2 {
            # "Load enabled"
            n150 = Build Array (concatenate)(w358, w357) -> (w361:waveform(dbl)[])
            n151 = Build Array (concatenate)(w360, w359) -> (w362:waveform(dbl)[])
          }
          frame 3, Default {
            # "Source and load enabled"
            n152 = Build Array (concatenate)(w372, w371, w366, w365) -> (w370:waveform(dbl)[])
            n153 = Build Array (concatenate)(w368, w369, w364, w363) -> (w367:waveform(dbl)[])
          }
        }
        "VoltageGraph" <- w293
        "CurrentGraph" <- w292
        n154 = case shown="3, Default" w282 {
          tunnel: [w338 w340 w344] -> w287
          frame 1 {
            # "Source enabled"
            n155 = property on="PPSResourceNames" class="Arr (strict)"() -> ("Value"=w335:refnum<k15>[])  [unwired: 2 in, 2 out]
            n156 = Insert Into Array(array=w335, index=0, new element="SystemSource" ("string")) -> (w338:refnum<k15>[])
          }
          frame 2 {
            # "Load enabled"
            n157 = property on="LoadResourceNames" class="Arr (strict)"() -> ("Value"=w339:refnum<k15>[])  [unwired: 2 in, 2 out]
            n158 = Insert Into Array(array=w339, index=0, new element="SystemLoad" ("string")) -> (w340:refnum<k15>[])
          }
          frame 3, Default {
            # "Source and load enabled"
            n159 = property on="PPSResourceNames" class="Arr (strict)"() -> ("Value"=w348:refnum<k15>[])  [unwired: 2 in, 2 out]
            n160 = property on="LoadResourceNames" class="Arr (strict)"() -> ("Value"=w347:refnum<k15>[])  [unwired: 2 in, 2 out]
            n161 = Build Array("SystemSource" ("string"), "SystemLoad" ("string")) -> (w343:string[])
            n162 = Build Array (concatenate)(w348, w347) -> (w345:refnum<k15>[])
            n163 = Insert Into Array(array=w345, index=0, new element=w343) -> (w344:refnum<k15>[])
          }
        }
        n164 = control-ref of="VoltageGraph"() -> (w308:refnum<vi>)
        n165 = control-ref of="CurrentGraph"() -> (w307:refnum<vi>)
        n166 = Array Size(array=w287) -> (size(s)=w289:i32)
        n167 = Less?(x=w289, y=w290) -> (x < y?=w291:bool)
        n168 = Subtract(x=w290, y=w289) -> (x-y=w288:i32)
        n169 = case shown="True" w291 {
          tunnel: w288 -> [_ w333]
          tunnel: w287 -> [w329 w331]
          tunnel: [w329 w330] -> w286
          frame False {
            # "Pass firectly if more than 16"
          }
          frame True {
            # "Adding space if less than 16 char for better label visible"
            n170 = Initialize Array("" ("string"), w333) -> (w332:string[])
            n171 = Insert Into Array(array=w331, new element=w332) -> (w330:refnum<k15>[])  [unwired: 1 in]
          }
        }
        n172 = Build Array(w308, w307) -> (w306:refnum<vi>[])
        n173 = for {
          tunnel: w306 -> [w374] mode=indexing
          tunnel: w286 -> [w373]
          n174 = for {
            tunnel: w374 -> [w377]
            tunnel: w373 -> [w376] mode=indexing
            i -> [w375]
            n175 = property on="Property Node" class="WFGraph (strict)"(reference=w377, "Active Plot"=w375, "Plot.Plot Name"=w376) -> ()  [unwired: 1 in, 2 out]
          }
        }
      }
      frame "UpdateTable" {
        # "Add the values from measurement results to table"
        n176 = local read "Source enable/disable"() -> (w404:bool)
        n177 = local read "Load enable/disable"() -> (w405:bool)
        n178 = case shown="1006" "Load output function" {
          tunnel: [w450 w451] -> w423
          tunnel: "Load current/voltage limit range" -> [w450 w452]
          tunnel: "Load voltage/current level range" -> [w449 w451]
          tunnel: [w449 w452] -> w422
          frame 1007, Default {
            # "DC Current"
          }
          frame 1006 {
            # "DC Voltage"
          }
        }
        n179 = case shown="1006, Default" "Power ON/Source output function" {
          tunnel: [w454 w455] -> w429
          tunnel: "Source voltage/current level range" -> [w454 w456]
          tunnel: "Power ON/Source current/voltage limit range" -> [w453 w455]
          tunnel: [w453 w456] -> w426
          frame 1006, Default {
            # "DC Voltage"
          }
          frame 1007 {
            # "DC Current"
          }
        }
        n180 = Build Array(w404, w405) -> (w406:bool[])
        n181 = Boolean Array To Number(Boolean array=w406) -> (number=w403:u32)
        n182 = Build Array(w429, w426) -> (w421:dbl[])
        n183 = Build Array(w423, w422) -> (w420:dbl[])
        n184 = case shown="1" w403 {
          tunnel: w421 -> [_ w433 _ w439]
          tunnel: w420 -> [_ _ w435 w438]
          tunnel: [_ w433 w435 w437] -> w417
          tunnel: [_ string[] ["Source Voltage (V)", "Source Current (A)"] string[] ["Load Voltage (V)", "Load Current (A)"] string[] ["Source Voltage (V)", "Source Current (A)", "Load Voltage (V)", "Load Current (A)"]] -> w407
          frame 0, Default {
          }
          frame 1 {
            # "Source enabled"
          }
          frame 2 {
            # "Load enabled"
          }
          frame 3 {
            # "Source and load enabled"
            n185 = Build Array (concatenate)(w439, w438) -> (w437:dbl[])
          }
        }
        n186 = local read "Maximum values"() -> (w411:dbl[])
        n187 = local read "Minimum values"() -> (w412:dbl[])
        n188 = local read "Mean values"() -> (w413:dbl[])
        n189 = for {
          tunnel: [w448] -> w415 mode=indexing
          tunnel: w417 -> [w447] mode=indexing
          tunnel: "%.5f" ("initial string") -> [w443]
          tunnel: w413 -> [w446] mode=indexing
          tunnel: w412 -> [w445] mode=indexing
          tunnel: w411 -> [w444] mode=indexing
          tunnel: [w442] -> w410 mode=indexing
          tunnel: [w441] -> w409 mode=indexing
          tunnel: [w440] -> w408 mode=indexing
          n190 = Format Into String(format string=w443, w447) -> (resulting string=w448:string)  [unwired: 2 in, 1 out]
          n191 = Format Into String(format string=w443, w445) -> (resulting string=w441:string)  [unwired: 2 in, 1 out]
          n192 = Format Into String(format string=w443, w444) -> (resulting string=w440:string)  [unwired: 2 in, 1 out]
          n193 = Format Into String(format string=w443, w446) -> (resulting string=w442:string)  [unwired: 2 in, 1 out]
        }
        n194 = Build Array(w407, w415, w410, w409, w408) -> (w414:string[][])
        n195 = Transpose 2D Array(2D array=w414) -> (transposed array=→"Meas Table":string[][])
      }
      frame "Exit" {
        # "This case is triggered to close the User Interface from framework"
        n196 = Flush Queue(queue=w461, error in (no error)=w463) -> (queue out=w460:refnum<queue>, error out=w459:errorcluster)  [unwired: 1 out]
        n197 = Release Queue(queue=w460, force destroy? (F)=TRUE, error in (no error)=w459) -> (error out=w458:errorcluster)  [unwired: 2 out]
      }
      frame "Handle Error" {
        # "Handles errors"
      }
    }
  }
